vi "Length of string_0.vi"() -> ()   [LabVIEW 2015]
panel:
  in  "stop":bool
  in  "Tab Control":enum32{"Page 1", "Page 2"}(tab)
  in  "String":string
  out "String 2":string
  out "length":i32
  # "Length of string"
  # "Pardeep Kumar"
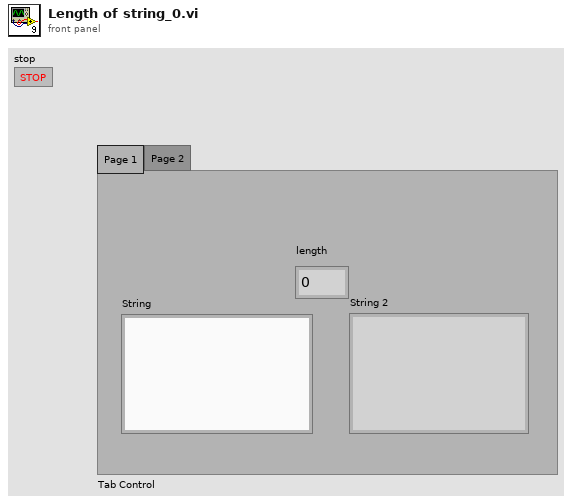
[diagram p1: front panel]
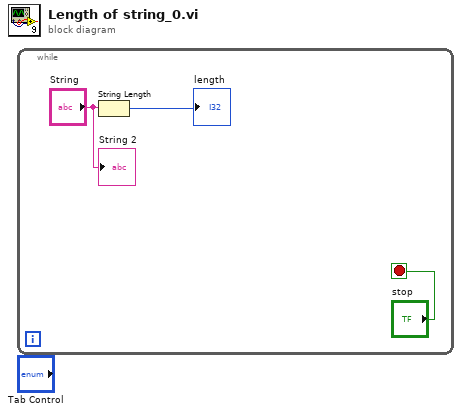
[diagram p0: block diagram]
diagram:
  n1 = while {
    stop <- "stop" stop-if-true
    n2 = String Length(string="String") -> (length=→"length":i32)
    "String 2" <- "String"
  }
